vi "Rx Core 2945 2955.vi"(0 "rx.ddc parameters":T1[](array[typedef]) {"if frequency shift" format="%#.48g"; "frequency shift" format="%#.48g"}, 1 "rx.reset":bool=TRUE, 2 "fifo 0":refnum<k21>, 3 "fifo 1":refnum<k21>, 5 "rx.samples to acquire":u32, 7 "rx.abort":bool, 9 "rx.stream enable":bool[](array[boolean]), 11 "rx.start trigger":bool, 12 "fifo 2":refnum<k21>, 13 "fifo 3":refnum<k21>) -> (4 "rx.state":T3, 6 "rx.samples processed":u32, 8 "rx.number of fifo overflows":u32, 10 "rx.number of iq data overflows":u64[](array[numeric]), 14 "rx.dsp reset done":bool)   [LabVIEW 2021]
uses:
  Stream Control State.ctl
  DDC Parameters 2945 2955.ctl
  <instrlib>/_niInstr/DSP/v1/Shared/Public/IQ Impairments.ctl
  <vilib>/rvi/eio/common/nirviEmuTemplateMethod_errors.vi
  <instrlib>/_niInstr/DSP/v1/FPGA/Public/Sub VIs/Data Conversion/I16 to IQ - 1 spc - S18.1.vi
  <vilib>/eio/EIONode/EIONode.xnode
  <instrlib>/_niInstr/Basic Elements/v1/FPGA/niInstr Basic Elements v1 FPGA.lvlib
  <instrlib>/_niInstr/DSP/v1/FPGA/niInstr DSP v1 FPGA.lvlib
  <instrlib>/_niInstr/DSP/v1/Shared/niInstr DSP v1 Shared.lvlib
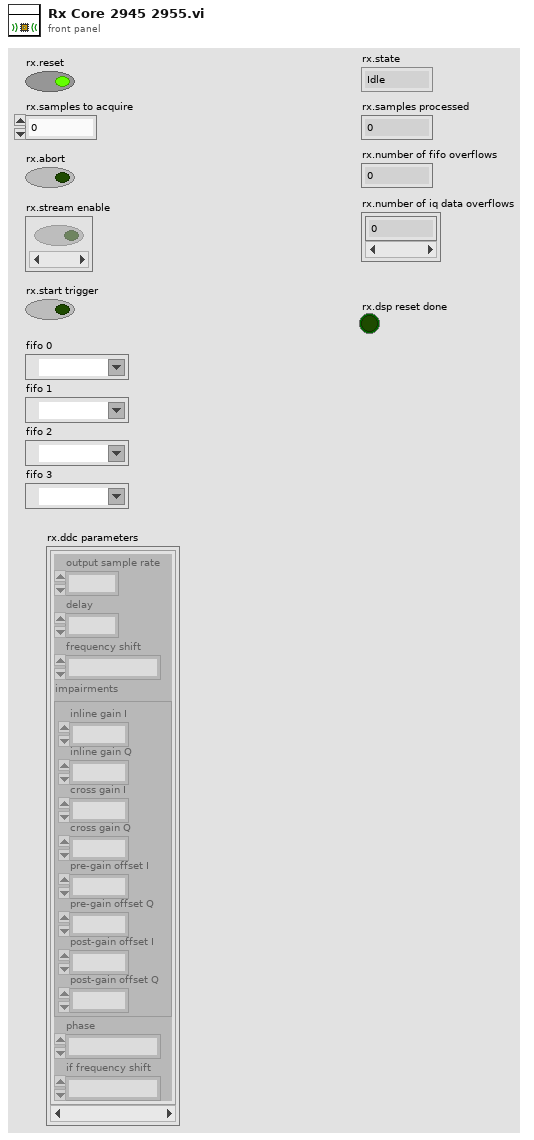
[diagram p1: front panel]
types:
  T1 = typedef "DDC Parameters 2945 2955.ctl" = cluster{"output sample rate":fxp<+,48,1>, "delay":fxp<+/-,16,0>, "frequency shift":fxp<+/-,48,0>, "impairments":T2, "phase":fxp<+/-,21,0>, "if frequency shift":fxp<+/-,48,0>}
  T2 = typedef "niInstr DSP v1 Shared.lvlib/IQ Impairments.ctl" = cluster{"inline gain I":fxp<+/-,18,1>, "inline gain Q":fxp<+/-,18,1>, "cross gain I":fxp<+/-,18,1>, "cross gain Q":fxp<+/-,18,1>, "pre-gain offset I":fxp<+/-,18,1>, "pre-gain offset Q":fxp<+/-,18,1>, "post-gain offset I":fxp<+/-,18,1>, "post-gain offset Q":fxp<+/-,18,1>}
  T3 = typedef "Stream Control State.ctl" = enum16{"Idle", "Active"}
  T4 = typedef "niInstr DSP v1 Shared.lvlib/IQ Data.ctl" = cluster{"I":fxp<+/-,18,1>, "Q":fxp<+/-,18,1>, "overflow":bool}
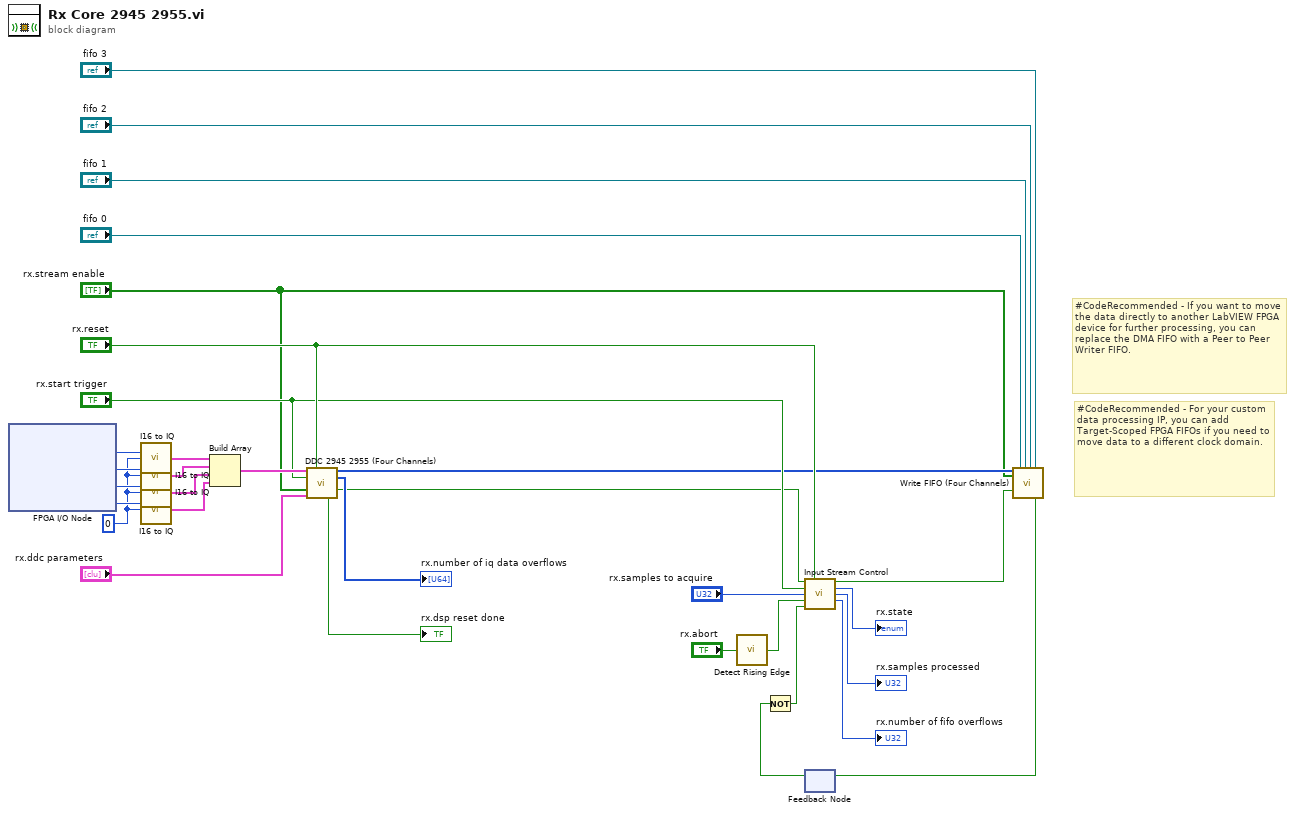
[diagram p0: block diagram]
diagram:
  w18 = i16 0 ("Q")
  # "#CodeRecommended - For your custom data processing IP, you can add Target-Scoped FPGA FIFOs if you need to move data to a different clock domain."
  # "#CodeRecommended - If you want to move the data directly to another LabVIEW FPGA device for further processing, you can replace the DMA FIFO with a Peer to Peer Writer FIFO."
  n1 = xnode "FPGA I/O Node"() -> ("RF 0/Rx/Rx1"=w22:i16, "RF 0/Rx/Rx2"=w21:i16, "RF 1/Rx/Rx1"=w20:i16, "RF 1/Rx/Rx2"=w19:i16)  [unwired: 4 in, 4 out]
  n2 = call-poly <instrlib>:"I16 to IQ.vi"("I"=w22, "Q"=w18) -> ("IQ"=w31:T4)  [unwired: 13 in]
  n3 = call-poly <instrlib>:"I16 to IQ.vi"("I"=w21, "Q"=w18) -> ("IQ"=w32:T4)  [unwired: 13 in]
  n4 = call-poly <instrlib>:"I16 to IQ.vi"("I"=w20, "Q"=w18) -> ("IQ"=w16:T4)  [unwired: 13 in]
  n5 = call-poly <instrlib>:"I16 to IQ.vi"("I"=w19, "Q"=w18) -> ("IQ"=w17:T4)  [unwired: 13 in]
  n6 = Build Array(w31, w32, w16, w17) -> (w9:T4[])
  n7 = call "DDC 2945 2955 (Four Channels).vi"("data in"=w9, "reset"="rx.reset", "start trigger"="rx.start trigger", "enable"="rx.stream enable", "ddc parameters"="rx.ddc parameters") -> ("data out"=w5:u32[], "number of overflows"=→"rx.number of iq data overflows":u64[], "output valid"=w3:bool, "dsp reset done"=→"rx.dsp reset done":bool)  [unwired: 7 in]
  n8 = call <instrlib>:"Detect Rising Edge.vi"("signal"="rx.abort") -> ("edge detected"=w30:bool)  [unwired: 14 in]
  n9 = feedback #1() -> (w23:bool)  [unwired: 1 in]
  n10 = Not(x=w23) -> (.not. x?=w27:bool)
  n11 = call "Input Stream Control.vi"("input valid"=w3, "reset"="rx.reset", "start trigger"="rx.start trigger", "burst size"="rx.samples to acquire", "abort"=w30, "fifo timeout"=w27) -> ("write stream"=w13:bool, "state"=→"rx.state":T3, "samples processed"=→"rx.samples processed":u32, "number of overflows"=→"rx.number of fifo overflows":u32)  [unwired: 5 in, 1 out]
  n12 = call "Write FIFO (Four Channels).vi"("data in"=w5, "enable"="rx.stream enable", "input valid"=w13, "fifo 0"="fifo 0", "fifo 1"="fifo 1", "fifo 2"="fifo 2", "fifo 3"="fifo 3") -> ("ready for input"=w12:bool)  [unwired: 12 in]
  n13 = feedback-in #1(w12) -> ()
